vi "parese_two_byte.vi"(11 "write buffer 2":string="00.00.00.00.00.00.00.00.00.00.00.00.00.00.00.00.00.00.00.00.%") -> (0 "x+y":u16)   [LabVIEW 2020]
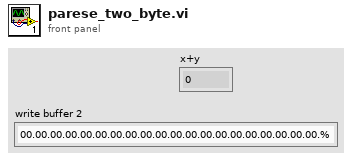
[diagram p1: front panel]
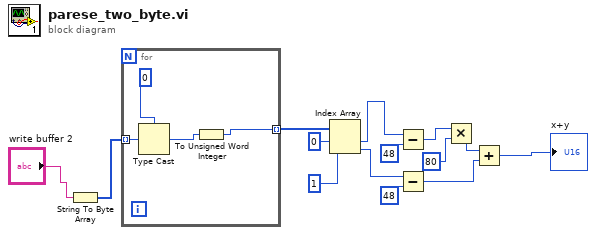
[diagram p0: block diagram]
diagram:
  n1 = String To Byte Array(string="write buffer 2") -> (unsigned byte array=w13:u8[])
  n2 = for {
    tunnel: w13 -> [w17] mode=indexing
    tunnel: [w15] -> w12 mode=indexing
    n3 = Type Cast(type=u8 0, x=w17) -> (*(type *) &x=w16:u8)
    n4 = To Unsigned Word Integer(number=w16) -> (unsigned 16bit integer=w15:u16)
  }
  n5 = Index Array(array=w12, index #1=0 ("index"), index #2=1 ("index")) -> (element #1=w9:u16, element #2=w6:u16)
  n6 = Subtract(x=w9, y=u8 48) -> (x-y=w1:u16)
  n7 = Subtract(x=w6, y=u8 48) -> (x-y=w5:u16)
  n8 = Multiply(x=w1, y=u8 80) -> (x*y=w3:u16)
  n9 = Add(x=w3, y=w5) -> (x+y=→"x+y":u16)
